vi "SVMDense_Crossvalidation_FromFile.vi"(8 "error in (no error)":errorcluster) -> (0 "error out":errorcluster, 3 "Predicted labels":dbl[](array[numeric]))   [LabVIEW 2015]
uses:
  LibSVM Sparse/Controls/Kernel.ctl
  LibSVM Sparse/Wrapper API/Controls/svm_kernel_type.ctl
  LibSVM Sparse/Controls/Options Training.ctl
  LibSVM Sparse/Controls/Parameters C_SVC.ctl
  Tools/Controls/Binary_ConfusionMatrix.ctl
  SubVIs/SVM Dense Cross-Validate C_SVC.vi
  Tools/SubVIs/Dense - Scale Problem Linear.vi
  Wrapper API/svmdense_cross_validation.vi
panel:
  out "Binary Confusion Matrix":T1
  in  "Param":T2={"C"=1.0, "weight_label"=[], "weight"=[]}
  in  "Nr Fold":i32=5 caption="Nr fold (LOO)"
  in  "Options":T3={"cache_size"=500.0, "eps"=0.001, "shrinking"=TRUE, "probability"=FALSE}
  in  "Kernel":T4
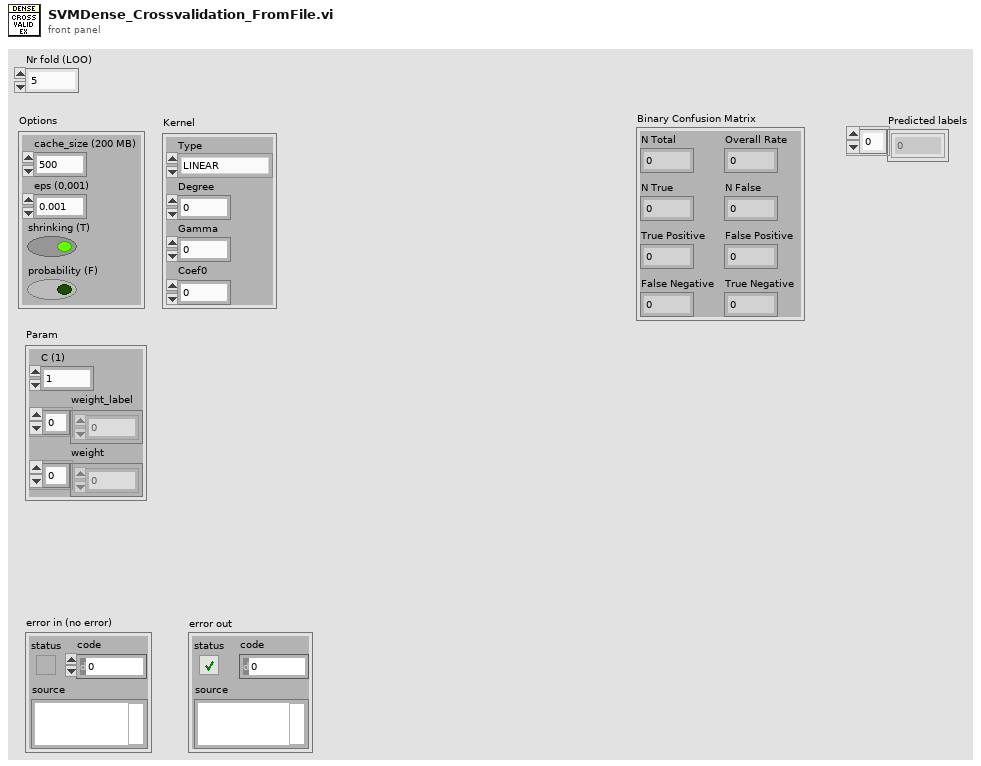
[diagram p1: front panel]
types:
  T1 = typedef "Binary_ConfusionMatrix.ctl" = cluster{"N Total":u32, "N True":u32, "N False":u32, "Overall Rate":dbl, "True Positive":dbl, "False Positive":dbl, "False Negative":dbl, "True Negative":dbl}
  T2 = typedef "Parameters C_SVC.ctl" = cluster{"C":dbl, "weight_label":i32[], "weight":dbl[]}
  T3 = typedef "Options Training.ctl" = cluster{"cache_size":dbl, "eps":dbl, "shrinking":bool, "probability":bool}
  T4 = typedef "Kernel.ctl" = cluster{"Type":T5, "Degree":i32, "Gamma":dbl, "Coef0":dbl}
  T5 = typedef "svm_kernel_type.ctl" = enum32{"LINEAR", "POLY", "RBF", "SIGMOID", "PRECOMPUTED"}
  T6 = typedef "svm_problem.ctl" = cluster{"y":dbl[], "x":cluster{T7[]}[]}
  T7 = typedef "svm_node.ctl" = cluster{"index":i32, "value":dbl}
  T8 = typedef "svmdense_problem.ctl" = cluster{"Y":dbl[], "X":cluster{"x":dbl[]}[]}
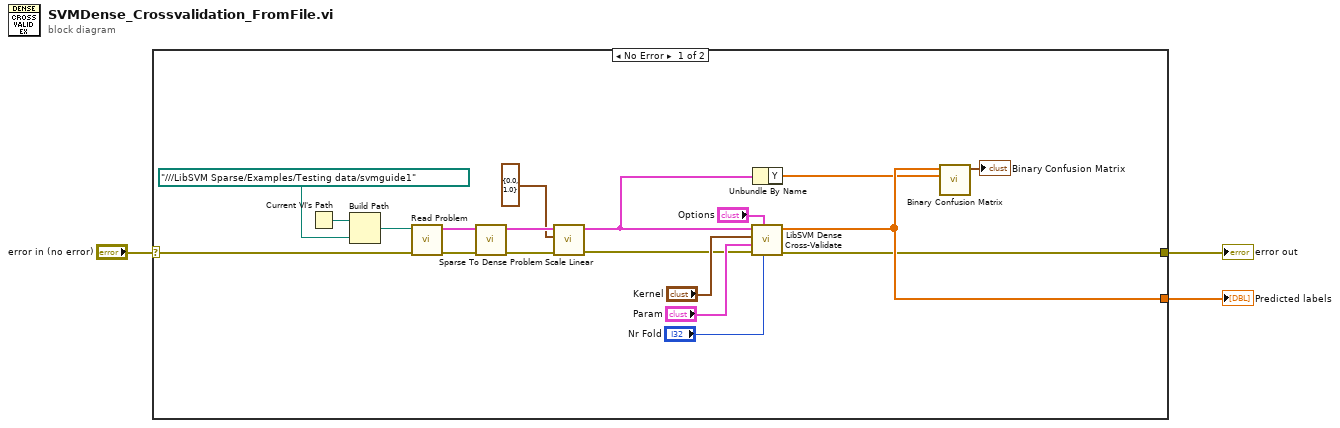
[diagram p0: block diagram]
diagram:
  n1 = case shown="No Error" "error in (no error)" {
    selector: "error in (no error)" -> [w14 w23]
    tunnel: [w5 w23] -> w1
    tunnel: [w13 _] -> w2
    frame No Error {
      n2 = Current VI's Path() -> (path=w21:path)
      n3 = Build Path(base path=w21, name or relative path=path "../../../LibSVM Sparse/Examples/Testing data/svmguide1") -> (appended path=w22:path)
      n4 = call "Read Problem.vi"("error in (no error)"=w14, "file path (use dialog)"=w22) -> ("error out"=w16:errorcluster, "svm_problem"=w15:T6)  [unwired: 8 in]
      n5 = call "Sparse To Dense Problem.vi"("error in (no error)"=w16, "Sparse Problem"=w15) -> ("error out"=w10:errorcluster, "Dense Problem"=w9:T8)  [unwired: 8 in]
      n6 = call-poly "Scale Linear.vi"("error in (no error)"=w10, "X Scaling limits"=cluster{"X lower":dbl, "X upper":dbl} {"X lower"=0.0, "X upper"=1.0}, "Problem"=w9) -> ("error out"=w7:errorcluster, "Scaled problem"=w6:T8)  [unwired: 6 in, 1 out]
      n7 = call-poly "LibSVM Dense Cross-Validate.vi"("Nr fold"="Nr Fold", "Options"="Options", "error in (no error)"=w7, "Param C_SVC"="Param", "Kernel"="Kernel", "Dense problem"=w6) -> ("error out"=w5:errorcluster, "Target"=w13:dbl[])  [unwired: 4 in]
      n8 = Unbundle By Name(w6) -> ("Y"=w12:dbl[])
      n9 = call "Binary Confusion Matrix.vi"("Actual Labels"=w12, "Predicted Labels"=w13) -> ("Binary Confusion Matrix"=→"Binary Confusion Matrix":T1)  [unwired: 8 in, 1 out]
    }
    frame Error {
    }
  }
  "Predicted labels" <- w2
  "error out" <- w1
